vi "Periodic Tasks.vi"(8 "error in":errorcluster) -> ()   [LabVIEW 2012]
doc: "This VI runs in parallel to other tasks. It can contain as many user-defined periodic loops as you need. These can carry out PID or other sorts of timed response."
uses:
  <vilib>/Rock Robotics/WPI/Solenoid/WPI_SolenoidValue.ctl
  <vilib>/Rock Robotics/SystemInterfaces/Utilities/FPGA_UtilitiesLED Source.ctl
  <vilib>/Rock Robotics/SystemInterfaces/Utilities/FPGA_UtilitiesLED State.ctl
  Robot Global Data.vi
  SubVI/Global 1 (shooter controls).vi
  <vilib>/Rock Robotics/WPI/Solenoid/WPI_SolenoidSetEnum.vi
  <vilib>/Rock Robotics/WPI/Joystick/WPI_JoystickGetSetRefNum.vi
  <vilib>/Rock Robotics/WPI/Compressor/WPI_CompressorGetSetRefNum.vi
  <vilib>/Rock Robotics/WPI/RobotDrive/WPI_RobotDriveGetSetRefNum.vi
  SubVI/Grabber States.ctl
  SubVI/grabber control buttons.vi
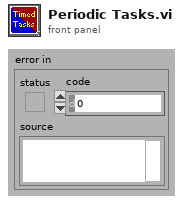
[diagram p1: front panel]
types:
  T1 = typedef "WPI_SolenoidDevRef.ctl" = cluster{"DevStatus":errorcluster, "Solenoid Module":T2, "Forward Solenoid Channel":T3, "Reverse Solenoid Channel":T3}
  T2 = typedef "FPGA_TypedefSolenoidModule.ctl" = enum16{"Solenoid Module 1", "Solenoid Module 2"}
  T3 = typedef "WPI_SolenoidChannel.ctl" = enum8{"Solenoid 1", "Solenoid 2", "Solenoid 3", "Solenoid 4", "Solenoid 5", "Solenoid 6", "Solenoid 7", "Solenoid 8", "Invalid"}
  T4 = typedef "WPI_AnalogChannelDevRef.ctl" = cluster{"DevStatus":errorcluster, "Analog Module":T5, "Analog Channel":T6}
  T5 = typedef "FPGA_TypedefAnalogModule.ctl" = enum16{"Analog Module 1", "Analog Module 2"}
  T6 = typedef "FPGA_AIChannel.ctl" = enum8{"AI 1", "AI 2", "AI 3", "AI 4", "AI 5", "AI 6", "AI 7", "AI 8", "Invalid"}
  T7 = typedef "WPI_SolenoidValue.ctl" = enum16{"Off", "On", "Forward", "Reverse"}
  T8 = typedef "WPI_JoystickDevRef.ctl" = cluster{"Device":T9}
  T9 = typedef "WPI_JoystickDeviceEnum.ctl" = enum16{"USB 1", "USB 2", "USB 3", "USB 4", "Kinect 1", "Kinect 2"}
  T10 = typedef "WPI_RobotDriveDevRef.ctl" = cluster{"DevStatus":errorcluster, "Motors[]":T11[], "Square Inputs":bool, "Max Output":dbl, "Isochronous":bool}
  T11 = typedef "WPI_MotorControlDeviceRef.ctl" = cluster{"DeviceStatus":errorcluster, "Type":enum16{"PWM", "CAN"}, "PWM":cluster{"Digital Module":T12, "PWM Channel":T13, "DeadBand":T14}, "CAN":cluster{"Device Number":u8, "Control Mode":T15, "Semaphore":T16, "Max Vout":dbl}, "Invert":bool, "TransformRef":T17, "InvTransformRef":T17}
  T12 = typedef "FPGA_TypedefDigitalModule.ctl" = enum16{"Digital Module 1", "Digital Module 2"}
  T13 = typedef "FPGA_DIOPWMChannel.ctl" = enum8{"PWM 1", "PWM 2", "PWM 3", "PWM 4", "PWM 5", "PWM 6", "PWM 7", "PWM 8", "PWM 9", "PWM 10", "Invalid"}
  T14 = typedef "WPI_PWMDeadband.ctl" = cluster{"Name":string, "maxPositivePwm":i32, "minPositivePwm":i32, "centerPwm":i32, "maxNegativePwm":i32, "minNegativePwm":i32, "angularRange":u16}
  T15 = typedef "WPI_CANJaguar_ControlMode.ctl" = enum8{"Percent VBus", "Current", "Speed", "Position", "Voltage"}
  T16 = typedef "Semaphore RefNum" = refnum<k1>
  T17 = typedef "WPI_PWMTransform_ConPane.ctl" = refnum<vi>
  T18 = cluster{"JoystickDevRef":T8, "RobotDriveDevRef":T10}
  T19 = typedef "Grabber States.ctl" = enum16{"Ready", "Hunting", "Down", "Dropfrisbee"}
  T20 = typedef "WPI_DigitalInputDevRef.ctl" = cluster{"DevStatus":errorcluster, "DIO Channel":T21, "Digital Module":T12}
  T21 = typedef "FPGA_DIOChannel.ctl" = enum8{"DIO 1", "DIO 2", "DIO 3", "DIO 4", "DIO 5", "DIO 6", "DIO 7", "DIO 8", "DIO 9", "DIO 10", "DIO 11", "DIO 12", "DIO 13", "DIO 14", "Invalid"}
  T22 = cluster{"pickupoveride":bool, "stophunting?":bool, "wanthunt?":bool}
  T23 = enum16{"current", "add ", "subtract", "zero", "normal"}
  T24 = typedef "WPI_JoystickButtonState.ctl" = cluster{"Button 1":bool, "Button 2":bool, "Button 3":bool, "Button 4":bool, "Button 5":bool, "Button 6":bool, "Button 7":bool, "Button 8":bool, "Button 9":bool, "Button 10":bool, "Button 11":bool, "Button 12":bool}
  T25 = typedef "WPI_CompressorDevRef.ctl" = cluster{"DevStatus":errorcluster, "DigitalInputDevRef":T20, "RelayDevRef":T26}
  T26 = typedef "WPI_RelayDevRef.ctl" = cluster{"DevStatus":errorcluster, "Relay Channel":T27, "Digital Module":T12, "Relay Direction":T28}
  T27 = typedef "FPGA_DIORelayChannel.ctl" = enum8{"Relay 1", "Relay 2", "Relay 3", "Relay 4", "Relay 5", "Relay 6", "Relay 7", "Relay 8", "Invalid"}
  T28 = typedef "WPI_RelayDirection.ctl" = enum16{"Both directions", "Forward only", "Reverse only"}
  T29 = typedef "FPGA_UtilitiesLED State.ctl" = enum16{"Off", "On", "Toggle"}
  T30 = typedef "FPGA_UtilitiesLED Source.ctl" = enum16{"User LED", "FPGA LED"}
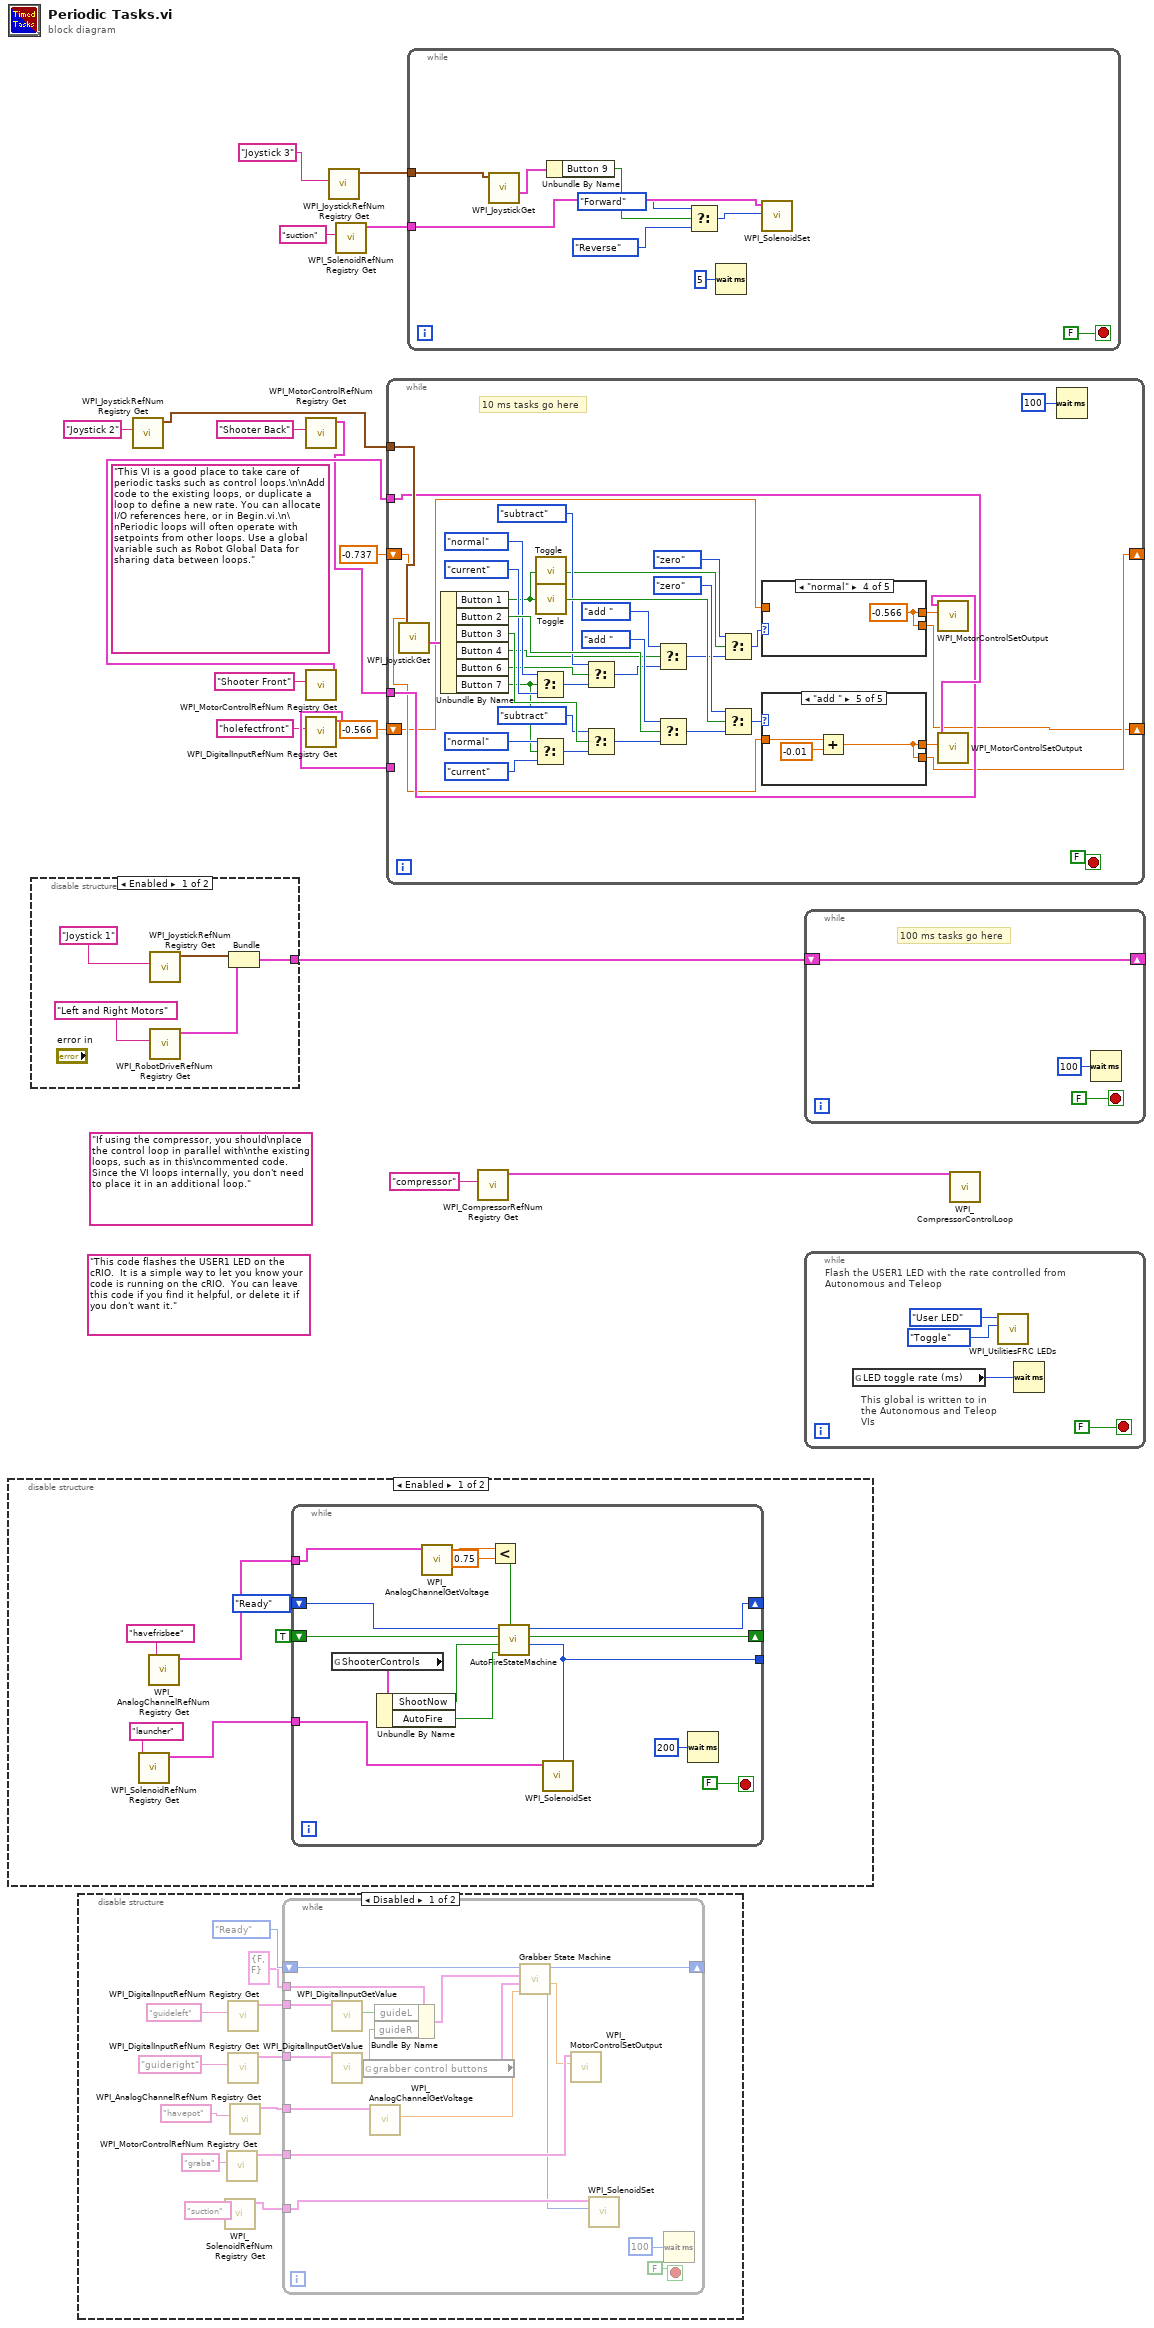
[diagram p0: block diagram]
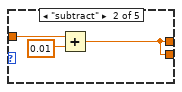
[diagram p6: hidden frame]
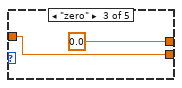
[diagram p7: hidden frame]
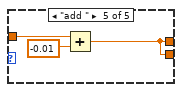
[diagram p8: hidden frame]
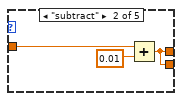
[diagram p10: hidden frame]
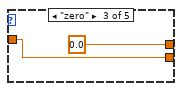
[diagram p11: hidden frame]
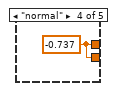
[diagram p12: hidden frame]
diagram:
  (unwired) "If using the compressor, you should\nplace the control loop in parallel with\nthe existing loops, such as in this\ncommented code. Since the VI loops internally, you don't need to place it in an additional loop."
  (unwired) "This code flashes the USER1 LED on the cRIO.  It is a simple way to let you know your code is running on the cRIO.  You can leave this code if you find it helpful, or delete it if you don't want it."
  (unwired) "This VI is a good place to take care of periodic tasks such as control loops.\n\nAdd code to the existing loops, or duplicate a loop to define a new rate. You can allocate I/O references here, or in Begin.vi.\n\nPeriodic loops will often operate with setpoints from other loops. Use a global variable such as Robot Global Data for sharing data between loops."
  n1 = disable-structure shown="Enabled" {
    frame Enabled {
      n2 = call <vilib>:"WPI_SolenoidRefNum Registry Get.vi"("refnum name"="launcher") -> ("SolenoidDevRef"=w22:T1)  [unwired: 9 in, 1 out]
      n3 = call <vilib>:"WPI_AnalogChannelRefNum Registry Get.vi"("refnum name"="havefrisbee") -> ("AIDeviceRef"=w20:T4)  [unwired: 9 in, 1 out]
      n4 = while {
        tunnel: [w36] -> _
        tunnel: w22 -> [w35]
        shift-right: [w34] -> _
        shift-left: enum16{"Ready", "Fire1", "Auto"}."Ready" ("NextState") -> [w33]
        shift-right: [w32] -> _
        shift-left: TRUE ("ShotComplete") -> [w31]
        tunnel: w20 -> [w27]
        stop <- FALSE stop-if-true
        n5 = global read "Global 1 (shooter controls).vi" "ShooterControls"() -> (w28:cluster{"ShootNow":bool, "AutoFire":bool})
        n6 = Unbundle By Name(w28) -> ("ShootNow"=w30:bool, "AutoFire"=w29:bool)
        n7 = call <vilib>:"WPI_AnalogChannelGetVoltage.vi"("AIDeviceRef"=w27) -> ("Voltage"=w26:dbl)  [unwired: 8 in, 2 out]
        n8 = Less?(x=w26, y=0.75) -> (x < y?=w25:bool)
        n9 = call "AutoFireStateMachine.vi"("FrisbeeInChamber"=w25, "AutoFire"=w29, "TriggerPulled"=w30, "LastShotComplete"=w31, "LastState"=w33) -> ("SolenoidState"=w36:T7, "ShotComplete"=w32:bool, "NextState"=w34:enum16{"Ready", "Fire1", "Auto"})  [unwired: 4 in]
        n10 = call-poly <vilib>:"WPI_SolenoidSet.vi"("Value"=w36, "SolenoidDevRef"=w35) -> ()  [unwired: 8 in, 2 out]
        n11 = Wait (ms)(milliseconds to wait=u32 200) -> ()  [unwired: 1 out]
      }
    }
    frame Disabled {
    }
  }
  n12 = disable-structure shown="Enabled" {
    disable-tunnel: [w39 _] -> w17
    frame Enabled {
      n13 = call <vilib>:"WPI_JoystickRefNum Registry Get.vi"("refnum name"="Joystick 1") -> ("JoystickDevRef"=w41:T8)  [unwired: 1 in, 9 out]
      n14 = call <vilib>:"WPI_RobotDriveRefNum Registry Get.vi"("refnum name"="Left and Right Motors") -> ("RobotDriveDevRef"=w40:T10)  [unwired: 1 in, 9 out]
      n15 = Bundle("JoystickDevRef"=w41, "RobotDriveDevRef"=w40) -> (w39:T18)  [unwired: 1 out]
    }
    frame Disabled {
    }
  }
  n16 = disable-structure shown="Disabled" {
    frame Disabled {
      n17 = call <vilib>:"WPI_SolenoidRefNum Registry Get.vi"("refnum name"="suction") -> ("SolenoidDevRef"=w47:T1)  [unwired: 9 in, 1 out]
      n18 = call <vilib>:"WPI_MotorControlRefNum Registry Get.vi"("refnum name"="graba") -> ("MotorControlDevRef"=w48:T11)  [unwired: 9 in, 1 out]
      n19 = call <vilib>:"WPI_DigitalInputRefNum Registry Get.vi"("refnum name"="guideleft") -> ("DigitalInputDevRef"=w50:T20)  [unwired: 9 in, 1 out]
      n20 = call <vilib>:"WPI_DigitalInputRefNum Registry Get.vi"("refnum name"="guideright") -> ("DigitalInputDevRef"=w51:T20)  [unwired: 9 in, 1 out]
      n21 = call <vilib>:"WPI_AnalogChannelRefNum Registry Get.vi"("refnum name"="havepot") -> ("AIDeviceRef"=w49:T4)  [unwired: 9 in, 1 out]
      n22 = while {
        shift-right: [w70] -> _
        shift-left: Grabber_States."Ready" ("Enum") -> [w69]
        tunnel: cluster{"guideL":bool, "guideR":bool} {"guideL"=FALSE, "guideR"=FALSE} ("Limit Switches") -> [w68]
        tunnel: w51 -> [w66]
        tunnel: w50 -> [w64]
        tunnel: w49 -> [w62]
        tunnel: w48 -> [w60]
        tunnel: w47 -> [w58]
        stop <- FALSE stop-if-true
        n23 = call <vilib>:"WPI_DigitalInputGetValue.vi"("DigitalInputDevRef"=w64) -> ("Value"=w63:bool)  [unwired: 8 in, 2 out]
        n24 = call <vilib>:"WPI_DigitalInputGetValue.vi"("DigitalInputDevRef"=w66) -> ("Value"=w65:bool)  [unwired: 8 in, 2 out]
        n25 = global read "grabber control buttons.vi" "grabber control buttons"() -> (w56:T22)
        n26 = call <vilib>:"WPI_AnalogChannelGetVoltage.vi"("AIDeviceRef"=w62) -> ("Voltage"=w61:dbl)  [unwired: 8 in, 2 out]
        n27 = Bundle By Name(cluster=w68, "guideL"=w63, "guideR"=w65) -> (w67:cluster{"guideL":bool, "guideR":bool})
        n28 = call "Grabber State Machine.vi"("location of arms"=w61, "grabber control buttons"=w56, "Limit Switches"=w67, "Laststate"=w69) -> ("suctioncup"=w57:T7, "Pickup Motor"=w59:dbl, "Next state"=w70:T19)  [unwired: 5 in]
        n29 = call <vilib>:"WPI_MotorControlSetOutput.vi"("Output"=w59, "MotorControlDevRef"=w60) -> ()  [unwired: 7 in, 3 out]
        n30 = call-poly <vilib>:"WPI_SolenoidSet.vi"("Value"=w57, "SolenoidDevRef"=w58) -> ()  [unwired: 8 in, 2 out]
        n31 = Wait (ms)(milliseconds to wait=u32 100) -> ()  [unwired: 1 out]
      }
    }
    frame Enabled {
    }
  }
  n32 = call <vilib>:"WPI_JoystickRefNum Registry Get.vi"("refnum name"="Joystick 2") -> ("JoystickDevRef"=w11:T8)  [unwired: 1 in, 9 out]
  n33 = call <vilib>:"WPI_MotorControlRefNum Registry Get.vi"("refnum name"="Shooter Back") -> ("MotorControlDevRef"=w9:T11)  [unwired: 9 in, 1 out]
  n34 = call <vilib>:"WPI_MotorControlRefNum Registry Get.vi"("refnum name"="Shooter Front") -> ("MotorControlDevRef"=w10:T11)  [unwired: 9 in, 1 out]
  n35 = call <vilib>:"WPI_DigitalInputRefNum Registry Get.vi"("refnum name"="holefectfront") -> ("DigitalInputDevRef"=w14:T20)  [unwired: 9 in, 1 out]
  n36 = call <vilib>:"WPI_JoystickRefNum Registry Get.vi"("refnum name"="Joystick 3") -> ("JoystickDevRef"=w3:T8)  [unwired: 1 in, 9 out]
  n37 = call <vilib>:"WPI_SolenoidRefNum Registry Get.vi"("refnum name"="suction") -> ("SolenoidDevRef"=w1:T1)  [unwired: 9 in, 1 out]
  n38 = while {
    tunnel: w14 -> [_]
    tunnel: w11 -> [w108]
    tunnel: w10 -> [w106]
    tunnel: w9 -> [w105]
    shift-right: [w79] -> _
    shift-left: -0.566 ("Output") -> [w73]
    shift-right: [w91] -> _
    shift-left: -0.737 ("Output") -> [w90]
    stop <- FALSE stop-if-true
    # "10 ms tasks go here"
    n39 = call <vilib>:"WPI_JoystickGet.vi"("JoystickDevRef"=w108) -> ("Buttons"=w107:T24)  [unwired: 4 in, 2 out]
    n40 = Unbundle By Name(w107) -> ("Button 1"=w77:bool, "Button 2"=w100:bool, "Button 3"=w97:bool, "Button 4"=w76:bool, "Button 6"=w75:bool, "Button 7"=w74:bool)
    n41 = Select(t=T23."normal", s=w74, f=T23."current") -> (s? t:f=w87:T23)
    n42 = Select(t=T23."normal", s=w74, f=T23."current") -> (s? t:f=w95:T23)
    n43 = call "Toggle.vi"("Boolean"=w77) -> ("Boolean 2"=w81:bool)
    n44 = call "Toggle.vi"("Boolean"=w77) -> ("Boolean 2"=w103:bool)
    n45 = Select(t=T23."subtract", s=w75, f=w87) -> (s? t:f=w85:T23)
    n46 = Select(t=T23."subtract", s=w97, f=w95) -> (s? t:f=w98:T23)
    n47 = Select(t=T23."add ", s=w76, f=w85) -> (s? t:f=w83:T23)
    n48 = Select(t=T23."add ", s=w100, f=w98) -> (s? t:f=w101:T23)
    n49 = Select(t=T23."zero", s=w81, f=w83) -> (s? t:f=w82:T23)
    n50 = Select(t=T23."zero", s=w103, f=w101) -> (s? t:f=w102:T23)
    n51 = case shown="\"normal\"" w82 {
      tunnel: [w111 w114 0.0 w117 w118] -> w78
      tunnel: [w111 w114 w115 w117 w118] -> w79
      tunnel: w73 -> [w111 w113 w115 _ w120]
      frame "current", Default {
      }
      frame "subtract" {
        n52 = Add(x=w113, y=0.01) -> (x+y=w114:dbl)
      }
      frame "zero" {
      }
      frame "normal" {
        w117 = -0.566 ("Output")
      }
      frame "add " {
        n53 = Add(x=w120, y=-0.01) -> (x+y=w118:dbl)
      }
    }
    n54 = case shown="\"add \"" w102 {
      tunnel: [w121 w124 0.0 w127 w128] -> w92
      tunnel: [w121 w124 w125 w127 w128] -> w91
      tunnel: w90 -> [w121 w123 w125 _ w130]
      frame "current", Default {
      }
      frame "subtract" {
        n55 = Add(x=w123, y=0.01) -> (x+y=w124:dbl)
      }
      frame "zero" {
      }
      frame "normal" {
        w127 = -0.737 ("Output")
      }
      frame "add " {
        n56 = Add(x=w130, y=-0.01) -> (x+y=w128:dbl)
      }
    }
    n57 = call <vilib>:"WPI_MotorControlSetOutput.vi"("Output"=w78, "MotorControlDevRef"=w105) -> ()  [unwired: 7 in, 3 out]
    n58 = call <vilib>:"WPI_MotorControlSetOutput.vi"("Output"=w92, "MotorControlDevRef"=w106) -> ()  [unwired: 7 in, 3 out]
    n59 = Wait (ms)(milliseconds to wait=u32 100) -> ()  [unwired: 1 out]
  }
  n60 = while {
    tunnel: w3 -> [w138]
    tunnel: w1 -> [w134]
    stop <- FALSE stop-if-true
    n61 = call <vilib>:"WPI_JoystickGet.vi"("JoystickDevRef"=w138) -> ("Buttons"=w137:T24)  [unwired: 4 in, 2 out]
    n62 = Unbundle By Name(w137) -> ("Button 9"=w133:bool)
    n63 = Select(t=WPI_SolenoidValue."Forward" ("Value"), s=w133, f=WPI_SolenoidValue."Reverse" ("Value")) -> (s? t:f=w135:T7)
    n64 = Wait (ms)(milliseconds to wait=u32 5) -> ()  [unwired: 1 out]
    n65 = call-poly <vilib>:"WPI_SolenoidSet.vi"("Value"=w135, "SolenoidDevRef"=w134) -> ()  [unwired: 8 in, 2 out]
  }
  n66 = call <vilib>:"WPI_CompressorRefNum Registry Get.vi"("refnum name"="compressor") -> ("CompressorDevRef"=w16:T25)  [unwired: 9 in, 1 out]
  n67 = while {
    shift-right: [w140] -> _
    shift-left: w17 -> [w140]
    stop <- FALSE stop-if-true
    # "100 ms tasks go here"
    n68 = Wait (ms)(milliseconds to wait=u32 100) -> ()  [unwired: 1 out]
  }
  n69 = while {
    stop <- FALSE stop-if-true
    # "This global is written to in the Autonomous and Teleop VIs"
    # "Flash the USER1 LED with the rate controlled from Autonomous and Teleop"
    n70 = global read "Robot Global Data.vi" "LED toggle rate (ms)"() -> (w143:u32)
    n71 = call <vilib>:"WPI_UtilitiesFRC LEDs.vi"("State"=FPGA_UtilitiesLED_State."Toggle", "LED Type"=FPGA_UtilitiesLED_Source."User LED") -> ()  [unwired: 1 in, 9 out]
    n72 = Wait (ms)(milliseconds to wait=w143) -> ()  [unwired: 1 out]
  }
  n73 = call <vilib>:"WPI_CompressorControlLoop.vi"("CompressorDevRef"=w16) -> ()  [unwired: 11 in]
